vi "HFRR ADV v07.vi"() -> ()   [LabVIEW 2025] (continued)
            n1283 = local read "TEMP"() -> (w1608:dbl)
            n1284 = local write "FF 3"(w1604) -> ()
            n1285 = Compound Arithmetic op=OR("FRICVALZ 4", "FRICVALZ 3", "FRICVALZ 2") -> (w1601:bool)
            n1286 = case shown="True" w1601 {
              tunnel: w1594 -> [_ w1615]
              frame False {
              }
              frame True {
                w1614 = FALSE ("FRICVALZ")
                n1287 = local write "FRICVALZ 3"(w1614) -> ()
                n1288 = local write "FRICVALZ 2"(w1614) -> ()
                n1289 = local write "FRICVALZ 4"(w1614) -> ()
                "FRICVALZ" <- w1615
              }
            }
            n1290 = Not A Number/Path/Refnum?(number/path/refnum=w1608) -> (NaN/Path/Refnum?=w1607:bool)
            n1291 = Not A Number/Path/Refnum?(number/path/refnum=w1604) -> (NaN/Path/Refnum?=w1606:bool)
            n1292 = Divide(x=w1604, y=1.96) -> (x/y=w1591:dbl)
            n1293 = Compound Arithmetic op=OR(w1607, w1606) -> (w1605:bool)
            n1294 = Not A Number/Path/Refnum?(number/path/refnum=w1591) -> (NaN/Path/Refnum?=w1602:bool)
            n1295 = case shown="True" w1605 {
              frame False {
              }
              frame True {
                n1296 = local write "TEMP"(0.0 ("TEMP")) -> ()
                n1297 = local write "FF 2"(0.0 ("FF 2")) -> ()
                n1298 = local write "reinit"(TRUE ("reinit")) -> ()
              }
            }
            n1299 = Select(t=0.0, s=w1602, f=w1591) -> (s? t:f=w1590:dbl)
            "COF 2" <- w1590
            n1300 = local write "COF 3"(w1590) -> ()
          }
        }
      }
    }
    n1301 = Wait (ms)(milliseconds to wait=u32 50) -> ()  [unwired: 1 out]
    n1302 = local read "Quit"() -> (w1530:bool)
    "Rate" <- 2500.0 ("No of Samples")
  }
  n1303 = VISA Close(VISA resource name=w52, error in (no error)=w51) -> (error out=w49:errorcluster)
  n1304 = call <vilib>:"Clear Errors.vi"("error in (no error)"=w49) -> ()  [unwired: 5 in, 2 out]
  n1305 = VISA Close(VISA resource name=w37, error in (no error)=w36) -> ()  [unwired: 1 out]
  n1306 = while {
    tunnel: w57 -> [_]
    tunnel: [w1642] -> _
    tunnel: [w1618] -> w56
    i -> [w1642]
    stop <- w1618 stop-if-true
    # "C:\\LAB-IQ-NXT\\Scar View.exe"
    n1307 = local read "OK Button 16"() -> (w1631:bool)
    n1308 = local read "Main Tab"() -> (w1624:T2)
    n1309 = local read "service 3"() -> (w1625:bool)
    n1310 = local read "OPEN 6"() -> (w1627:bool)
    n1311 = local read "EDIT 2"() -> (w1629:bool)
    n1312 = local read "RUN"() -> (w1639:bool)
    n1313 = local read "RUN"() -> (w1641:bool)
    n1314 = case shown="True" "EDIT 3" {
      frame False {
      }
      frame True {
        n1315 = local write "EDIT 3"(FALSE ("EDIT 3")) -> ()
        n1316 = local write "Main Tab"(T2."About" ("Main Tab")) -> ()
      }
    }
    n1317 = case shown="\"CEC F-096-A-06\"" "TEST STANDARD" {
      tunnel: [2.0 ("Set Temp") 0.0 ("Set Temp") 2.0 ("Set Temp") 0.0 ("Set Temp")] -> w1630
      frame "ASTM D6079", Default {
        w2183 = 50.0 ("Hz")
        w2184 = 53.0 ("Set Rh")
        w2186 = 1.0 ("Set Strk")
        w2185 = 60.0 ("Set Temp")
        # "astm hide"
        n1318 = local write "NORMAL LOAD"(200.0 ("NORMAL LOAD")) -> ()
        n1319 = local write "Set Strk"(w2186) -> ()
        n1320 = local write "Set Hz"(w2183) -> ()
        n1321 = local write "test time"(75.0 ("test time")) -> ()
        n1322 = local write "Set Rh"(w2184) -> ()
        n1323 = local write "Set Temp"(w2185) -> ()
        n1324 = local write "Set Stroke:"(w2186) -> ()
        n1325 = local write "Set Humidity:"(w2184) -> ()
        n1326 = local write "Set Frequency:"(w2183) -> ()
        n1327 = local write "Set Temperature:"(w2185) -> ()
        "Test Standard" <- "ASTM D6079" ("Test Standard 2")
      }
      frame "ISO 12156" {
        n1328 = local write "NORMAL LOAD"(200.0 ("NORMAL LOAD")) -> ()
        n1329 = local write "Set Strk"(1.0 ("Set Strk")) -> ()
        n1330 = local write "Set Hz"(50.0 ("Hz")) -> ()
        n1331 = local write "test time"(75.0 ("test time")) -> ()
        n1332 = local write "Set Rh"(53.0 ("Set Rh")) -> ()
        n1333 = local write "Set Temp"(60.0 ("Set Temp")) -> ()
      }
      frame "CEC F-096-A-06" {
        n1334 = local write "NORMAL LOAD"(200.0 ("NORMAL LOAD")) -> ()
        n1335 = local write "Set Strk"(1.0 ("Set Strk")) -> ()
        n1336 = local write "Set Hz"(50.0 ("Hz")) -> ()
        n1337 = local write "test time"(75.0 ("test time")) -> ()
        n1338 = local write "Set Rh"(53.0 ("Set Rh")) -> ()
        n1339 = local write "Set Temp"(60.0 ("Set Temp")) -> ()
      }
      frame "Custom" {
      }
    }
    n1340 = case shown="False" w1639 {
      frame False {
      }
      frame True {
      }
    }
    n1341 = Or(x=w1627, y=w1625) -> (x .or. y?=w1626:bool)
    n1342 = case shown="\"About\"" w1624 {
      tunnel: [T23."Acquire" ("Main Tab") T23."Compare Files" ("Main Tab") T23."About" ("Main Tab")] -> w1637
      frame "Acquire", Default {
      }
      frame "Compare Files" {
      }
      frame "About" {
      }
    }
    n1343 = Or(x=w1631, y="OPEN") -> (x .or. y?=w1632:bool)
    n1344 = case shown="True" w1632 {
      tunnel: w1631 -> [_ w1772]
      frame False {
      }
      frame True {
        n1345 = stacked-sequence {
          tunnel: w1772 -> [_ w1839 _ _]
          frame #0 {
            w1788 = "  " ("String 6")
            n1346 = local write "OPEN"(FALSE ("open")) -> ()
            n1347 = local read "string1 4"() -> (w1774:string)
            n1348 = local read "string1 3"() -> (w1775:string)
            n1349 = local read "string1 2"() -> (w1776:string)
            n1350 = local write "String 6"(w1788) -> ()
            n1351 = local write "String 7"(w1788) -> ()
            n1352 = local write "String 8"(w1788) -> ()
            n1353 = local write "String 12"(w1788) -> ()
            n1354 = property on="OPEN" class="Bool (strict)"("Visible"=FALSE) -> ()  [unwired: 2 in, 2 out]
            n1355 = local read "OK Button 16"() -> (w1773:bool)
            n1356 = String To Path(string=w1774) -> (path=w1782:path)
            n1357 = String To Path(string=w1775) -> (path=w1783:path)
            n1358 = String To Path(string=w1776) -> (path=w1784:path)
            n1359 = case shown="True" w1773 {
              tunnel: [w1789 w1790] -> w1777
              frame False {
                n1360 = local read "string1"() -> (w1789:string)
              }
              frame True {
                n1361 = local read "String Indicator 4"() -> (w1790:string)
              }
            }
            n1362 = Open/Create/Replace File "Open File"(file path (use dialog)=w1784) -> (refnum out=w1780:refnum<file>)  [unwired: 5 in, 2 out]
            n1363 = Open/Create/Replace File "Open File"(file path (use dialog)=w1783) -> (refnum out=w1779:refnum<file>)  [unwired: 5 in, 2 out]
            n1364 = Open/Create/Replace File "Open File"(file path (use dialog)=w1782) -> (refnum out=w1778:refnum<file>)  [unwired: 5 in, 2 out]
            n1365 = while {
              tunnel: w1780 -> [w1802]
              i -> [w1798]
              stop <- w1797 continue-if-true
              (unwired) TRUE ("line mode (F)")
              n1366 = Read from Text File "Read File"(file (use dialog)=w1802) -> (text=w1799:string)  [unwired: 3 in, 3 out]
              n1367 = local write "Numeric 11"(w1798) -> ()
              n1368 = String Length(string=w1799) -> (length=w1801:i32)
              n1369 = Greater?(x=w1801, y=1) -> (0:w1797:bool)
            }
            n1370 = while {
              tunnel: w1779 -> [w1808]
              i -> [w1804]
              stop <- w1803 continue-if-true
              (unwired) TRUE ("line mode (F)")
              n1371 = Read from Text File "Read File"(file (use dialog)=w1808) -> (text=w1805:string)  [unwired: 3 in, 3 out]
              n1372 = local write "Numeric 12"(w1804) -> ()
              n1373 = String Length(string=w1805) -> (length=w1807:i32)
              n1374 = Greater?(x=w1807, y=1) -> (0:w1803:bool)
            }
            n1375 = while {
              tunnel: w1778 -> [w1814]
              i -> [w1810]
              stop <- w1809 continue-if-true
              (unwired) TRUE ("line mode (F)")
              n1376 = Read from Text File "Read File"(file (use dialog)=w1814) -> (text=w1811:string)  [unwired: 3 in, 3 out]
              n1377 = local write "Numeric 13"(w1810) -> ()
              n1378 = String Length(string=w1811) -> (length=w1813:i32)
              n1379 = Greater?(x=w1813, y=1) -> (0:w1809:bool)
            }
            n1380 = String To Path(string=w1777) -> (path=w1785:path)
            n1381 = Open/Create/Replace File "Open File"(file path (use dialog)=w1785) -> (refnum out=w1781:refnum<file>)  [unwired: 5 in, 2 out]
            n1382 = while {
              tunnel: w1781 -> [w1796]
              i -> [w1792]
              stop <- w1791 continue-if-true
              (unwired) TRUE ("line mode (F)")
              n1383 = Read from Text File "Read File"(file (use dialog)=w1796) -> (text=w1793:string)  [unwired: 3 in, 3 out]
              n1384 = local write "Numeric 8"(w1792) -> ()
              n1385 = String Length(string=w1793) -> (length=w1795:i32)
              n1386 = Greater?(x=w1795, y=1) -> (0:w1791:bool)
            }
          }
          frame #1 {
            w1966 = FALSE ("ACTUAL   MERGE")
            # "Sample Temp"
            # "ECR"
            # "COF"
            # "Time\nCOF\nFF\nTemp"
            n1387 = case shown="True" w1839 {
              tunnel: [w1986 w1987] -> w1840
              frame False {
                n1388 = local read "string1"() -> (w1986:string)
              }
              frame True {
                n1389 = local read "String Indicator 4"() -> (w1987:string)
              }
            }
            n1390 = local read "string1 3"() -> (w1884:string)
            n1391 = String To Path(string=w1884) -> (path=w1982:path)
            n1392 = String To Path(string=w1840) -> (path=w1971:path)
            n1393 = local read "Numeric 12"() -> (w1968:i32)
            n1394 = local read "Numeric 8"() -> (w1970:i32)
            n1395 = local read "string1 4"() -> (w1883:string)
            n1396 = local read "string1 2"() -> (w1885:string)
            n1397 = Open/Create/Replace File "Open File"(file path (use dialog)=w1971) -> (refnum out=w1985:refnum<file>, error out=w1984:errorcluster)  [unwired: 5 in, 1 out]
            n1398 = Open/Create/Replace File "Open File"(file path (use dialog)=w1982) -> (refnum out=w1978:refnum<file>, error out=w1979:errorcluster)  [unwired: 5 in, 1 out]
            n1399 = for {
              N: w1968 -> [_]
              tunnel: w1979 -> [w2059]
              tunnel: w1978 -> [w2058]
              tunnel: [w2048] -> w1937 mode=indexing
              tunnel: [w2046] -> w1935 mode=indexing
              tunnel: [w2047] -> w1931 mode=indexing
              tunnel: w1966 -> [_]
              tunnel: [w2040] -> w1933 mode=indexing
              tunnel: [w2036] -> w1915 mode=indexing
              tunnel: [w2032] -> w1891 mode=indexing
              tunnel: [w2029] -> w1872 mode=indexing
              tunnel: [w2025] -> w1831 mode=indexing
              (unwired) 9 ("length (rest)")
              (unwired) 9 ("length (rest)")
              (unwired) TRUE ("line mode (F)")
              n1400 = Read from Text File "Read File"(file (use dialog)=w2058, error in=w2059) -> (text=w2026:string)  [unwired: 2 in, 3 out]
              n1401 = local write "String 8"(w2026) -> ()
              n1402 = String Subset(string=w2026, offset (0)=85) -> (substring=w2028:string)  [unwired: 1 in]
              n1403 = String Subset(string=w2026, offset (0)=25) -> (substring=w2030:string)  [unwired: 1 in]
              n1404 = String Subset(string=w2026, offset (0)=55, length (rest)=9 ("length (rest)")) -> (substring=w2034:string)
              n1405 = String Subset(string=w2026, offset (0)=45, length (rest)=9 ("length (rest)")) -> (substring=w2039:string)
              n1406 = String Subset(string=w2026, offset (0)=65, length (rest)=9 ("length (rest)")) -> (substring=w2045:string)
              n1407 = String Subset(string=w2026, offset (0)=35, length (rest)=9 ("length (rest)")) -> (substring=w2049:string)
              n1408 = String Subset(string=w2026, offset (0)=0, length (rest)=14 ("length (rest)")) -> (substring=w2052:string)
              n1409 = String Subset(string=w2026, offset (0)=15, length (rest)=9 ("length (rest)")) -> (substring=w2055:string)
              n1410 = Fract/Exp String To Number(string=w2028) -> (number=w2025:dbl)  [unwired: 3 in, 1 out]
              n1411 = Fract/Exp String To Number(string=w2030) -> (number=w2029:dbl)  [unwired: 3 in, 1 out]
              n1412 = Fract/Exp String To Number(string=w2034) -> (number=w2032:dbl)  [unwired: 3 in, 1 out]
              n1413 = Fract/Exp String To Number(string=w2039) -> (number=w2036:dbl)  [unwired: 3 in, 1 out]
              n1414 = Fract/Exp String To Number(string=w2045) -> (number=w2042:dbl)  [unwired: 3 in, 1 out]
              n1415 = Fract/Exp String To Number(string=w2049) -> (number=w2047:dbl)  [unwired: 3 in, 1 out]
              n1416 = Fract/Exp String To Number(string=w2052) -> (number=w2048:dbl)  [unwired: 3 in, 1 out]
              n1417 = Fract/Exp String To Number(string=w2055) -> (number=w2046:dbl)  [unwired: 3 in, 1 out]
              n1418 = Add(x=w2042, y=0.0) -> (x+y=w2040:dbl)
            }
            n1419 = for {
              N: w1970 -> [_]
              tunnel: w1985 -> [w2133]
              tunnel: w1984 -> [w2132]
              tunnel: [w2122] -> w1897 mode=indexing
              tunnel: [w2120] -> w1954 mode=indexing
              tunnel: [w2121] -> w1949 mode=indexing
              tunnel: w1966 -> [_]
              tunnel: [w2114] -> w1951 mode=indexing
              tunnel: [w2110] -> w1920 mode=indexing
              tunnel: [w2106] -> w1895 mode=indexing
              tunnel: [w2102] -> w1876 mode=indexing
              tunnel: [w2097] -> w1836 mode=indexing
              (unwired) TRUE ("line mode (F)")
              # "freq"
              # "Stroke"
              # "Time"
              # "CoF"
              # "Humidity"
              # "Temp"
              # "Air Temp"
              # "ECR"
              n1420 = Read from Text File "Read File"(file (use dialog)=w2133, error in=w2132) -> (text=w2098:string)  [unwired: 2 in, 3 out]
              n1421 = local write "String 6"(w2098) -> ()
              n1422 = String Subset(string=w2098, offset (0)=35, length (rest)=9 ("length (rest)")) -> (substring=w2123:string)
              n1423 = String Subset(string=w2098, offset (0)=0, length (rest)=14 ("length (rest)")) -> (substring=w2126:string)
              n1424 = String Subset(string=w2098, offset (0)=15, length (rest)=9 ("length (rest)")) -> (substring=w2129:string)
              n1425 = Fract/Exp String To Number(string=w2123) -> (number=w2121:dbl)  [unwired: 3 in, 1 out]
              n1426 = Fract/Exp String To Number(string=w2126) -> (number=w2122:dbl)  [unwired: 3 in, 1 out]
              n1427 = Fract/Exp String To Number(string=w2129) -> (number=w2120:dbl)  [unwired: 3 in, 1 out]
              n1428 = String Subset(string=w2098, offset (0)=85, length (rest)=9 ("length (rest)")) -> (substring=w2099:string)
              n1429 = String Subset(string=w2098, offset (0)=25, length (rest)=9 ("length (rest)")) -> (substring=w2105:string)
              n1430 = String Subset(string=w2098, offset (0)=55, length (rest)=9 ("length (rest)")) -> (substring=w2107:string)
              n1431 = String Subset(string=w2098, offset (0)=45, length (rest)=9 ("length (rest)")) -> (substring=w2113:string)
              n1432 = String Subset(string=w2098, offset (0)=65, length (rest)=9 ("length (rest)")) -> (substring=w2119:string)
              n1433 = Fract/Exp String To Number(string=w2105) -> (number=w2102:dbl)  [unwired: 3 in, 1 out]
              n1434 = Fract/Exp String To Number(string=w2099) -> (number=w2097:dbl)  [unwired: 3 in, 1 out]
              n1435 = Fract/Exp String To Number(string=w2107) -> (number=w2106:dbl)  [unwired: 3 in, 1 out]
              n1436 = Fract/Exp String To Number(string=w2113) -> (number=w2110:dbl)  [unwired: 3 in, 1 out]
              n1437 = Fract/Exp String To Number(string=w2119) -> (number=w2116:dbl)  [unwired: 3 in, 1 out]
              n1438 = Add(x=w2116, y=0.0) -> (x+y=w2114:dbl)
            }
            n1439 = String To Path(string=w1883) -> (path=w1977:path)
            n1440 = String To Path(string=w1885) -> (path=w1983:path)
            n1441 = local read "Numeric 11"() -> (w1967:i32)
            n1442 = local read "Numeric 13"() -> (w1969:i32)
            n1443 = Open/Create/Replace File "Open File"(file path (use dialog)=w1983) -> (refnum out=w1981:refnum<file>, error out=w1980:errorcluster)  [unwired: 5 in, 1 out]
            n1444 = Open/Create/Replace File "Open File"(file path (use dialog)=w1977) -> (refnum out=w1976:refnum<file>, error out=w1975:errorcluster)  [unwired: 5 in, 1 out]
            n1445 = for {
              N: w1969 -> [_]
              tunnel: w1976 -> [w2024]
              tunnel: w1975 -> [w2023]
              tunnel: [w2013] -> w1929 mode=indexing
              tunnel: [w2012] -> w1922 mode=indexing
              tunnel: w1966 -> [_]
              tunnel: [w2001] -> w1927 mode=indexing
              tunnel: [w2006] -> w1924 mode=indexing
              tunnel: [w2002] -> w1914 mode=indexing
              tunnel: [w1997] -> w1889 mode=indexing
              tunnel: [w1993] -> w1870 mode=indexing
              tunnel: [w1988] -> w1830 mode=indexing
              (unwired) 1.0 ("x")
              (unwired) TRUE ("line mode (F)")
              n1446 = Read from Text File "Read File"(file (use dialog)=w2024, error in=w2023) -> (text=w1989:string)  [unwired: 2 in, 3 out]
              n1447 = local write "String 12"(w1989) -> ()
              n1448 = String Subset(string=w1989, offset (0)=85, length (rest)=9 ("length (rest)")) -> (substring=w1991:string)
              n1449 = String Subset(string=w1989, offset (0)=25, length (rest)=9 ("length (rest)")) -> (substring=w1995:string)
              n1450 = String Subset(string=w1989, offset (0)=55, length (rest)=9 ("length (rest)")) -> (substring=w1999:string)
              n1451 = String Subset(string=w1989, offset (0)=45, length (rest)=9 ("length (rest)")) -> (substring=w2004:string)
              n1452 = String Subset(string=w1989, offset (0)=65, length (rest)=9 ("length (rest)")) -> (substring=w2007:string)
              n1453 = String Subset(string=w1989, offset (0)=35, length (rest)=9 ("length (rest)")) -> (substring=w2014:string)
              n1454 = String Subset(string=w1989, offset (0)=0, length (rest)=14 ("length (rest)")) -> (substring=w2017:string)
              n1455 = String Subset(string=w1989, offset (0)=15, length (rest)=9 ("length (rest)")) -> (substring=w2020:string)
              n1456 = Fract/Exp String To Number(string=w1991) -> (number=w1988:dbl)  [unwired: 3 in, 1 out]
              n1457 = Fract/Exp String To Number(string=w1995) -> (number=w1993:dbl)  [unwired: 3 in, 1 out]
              n1458 = Fract/Exp String To Number(string=w1999) -> (number=w1997:dbl)  [unwired: 3 in, 1 out]
              n1459 = Fract/Exp String To Number(string=w2004) -> (number=w2002:dbl)  [unwired: 3 in, 1 out]
              n1460 = Fract/Exp String To Number(string=w2007) -> (number=w2010:dbl)  [unwired: 3 in, 1 out]
              n1461 = Fract/Exp String To Number(string=w2014) -> (number=w2012:dbl)  [unwired: 3 in, 1 out]
              n1462 = Fract/Exp String To Number(string=w2017) -> (number=w2013:dbl)  [unwired: 3 in, 1 out]
              n1463 = Fract/Exp String To Number(string=w2020) -> (number=w2001:dbl)  [unwired: 3 in, 1 out]
              n1464 = Add(x=w2010, y=0.0) -> (x+y=w2006:dbl)
            }
            n1465 = for {
              N: w1967 -> [_]
              tunnel: w1981 -> [w2096]
              tunnel: w1980 -> [w2095]
              tunnel: [w2085] -> w1947 mode=indexing
              tunnel: [w2083] -> w1945 mode=indexing
              tunnel: [w2084] -> w1940 mode=indexing
              tunnel: w1966 -> [_]
              tunnel: [w2077] -> w1942 mode=indexing
              tunnel: [w2073] -> w1918 mode=indexing
              tunnel: [w2069] -> w1893 mode=indexing
              tunnel: [w2065] -> w1874 mode=indexing
              tunnel: [w2060] -> w1832 mode=indexing
              (unwired) TRUE ("line mode (F)")
              n1466 = Read from Text File "Read File"(file (use dialog)=w2096, error in=w2095) -> (text=w2061:string)  [unwired: 2 in, 3 out]
              n1467 = local write "String 7"(w2061) -> ()
              n1468 = String Subset(string=w2061, offset (0)=85, length (rest)=9 ("length (rest)")) -> (substring=w2064:string)
              n1469 = String Subset(string=w2061, offset (0)=25, length (rest)=9 ("length (rest)")) -> (substring=w2066:string)
              n1470 = String Subset(string=w2061, offset (0)=55, length (rest)=9 ("length (rest)")) -> (substring=w2072:string)
              n1471 = String Subset(string=w2061, offset (0)=45, length (rest)=9 ("length (rest)")) -> (substring=w2074:string)
              n1472 = String Subset(string=w2061, offset (0)=65, length (rest)=9 ("length (rest)")) -> (substring=w2078:string)
              n1473 = String Subset(string=w2061, offset (0)=35, length (rest)=9 ("length (rest)")) -> (substring=w2086:string)
              n1474 = String Subset(string=w2061, offset (0)=0, length (rest)=14 ("length (rest)")) -> (substring=w2089:string)
              n1475 = String Subset(string=w2061, offset (0)=15, length (rest)=9 ("length (rest)")) -> (substring=w2092:string)
              n1476 = Fract/Exp String To Number(string=w2064) -> (number=w2060:dbl)  [unwired: 3 in, 1 out]
              n1477 = Fract/Exp String To Number(string=w2066) -> (number=w2065:dbl)  [unwired: 3 in, 1 out]
              n1478 = Fract/Exp String To Number(string=w2072) -> (number=w2069:dbl)  [unwired: 3 in, 1 out]
              n1479 = Fract/Exp String To Number(string=w2074) -> (number=w2073:dbl)  [unwired: 3 in, 1 out]
              n1480 = Fract/Exp String To Number(string=w2078) -> (number=w2081:dbl)  [unwired: 3 in, 1 out]
              n1481 = Fract/Exp String To Number(string=w2086) -> (number=w2084:dbl)  [unwired: 3 in, 1 out]
              n1482 = Fract/Exp String To Number(string=w2089) -> (number=w2085:dbl)  [unwired: 3 in, 1 out]
              n1483 = Fract/Exp String To Number(string=w2092) -> (number=w2083:dbl)  [unwired: 3 in, 1 out]
              n1484 = Add(x=w2081, y=0.0) -> (x+y=w2077:dbl)
            }
            n1485 = Delete From Array(array=w1872, index=0) -> (array with subset deleted=w1845:dbl[])  [unwired: 1 in, 1 out]
            n1486 = Delete From Array(array=w1915, index=0) -> (array with subset deleted=w1903:dbl[])  [unwired: 1 in, 1 out]
            n1487 = Delete From Array(array=w1933, index=0) -> (array with subset deleted=w1934:dbl[])  [unwired: 1 in, 1 out]
            n1488 = Delete From Array(array=w1935, index=0) -> (array with subset deleted=w1908:dbl[])  [unwired: 1 in, 1 out]
            n1489 = call-poly <vilib>:"Mean.vi"("X"=w1908) -> ("mean"=→"КОФ3":dbl)  [unwired: 1 out]
            n1490 = call-poly <vilib>:"Mean.vi"("X"=w1903) -> ("mean"=→"CP3":dbl)  [unwired: 1 out]
            n1491 = call-poly <vilib>:"Mean.vi"("X"=w1845) -> ("mean"=→"КОФ2 4":dbl)  [unwired: 1 out]
            n1492 = Delete From Array(array=w1836, index=0) -> (array with subset deleted=w1823:dbl[])  [unwired: 1 in, 1 out]
            n1493 = Delete From Array(array=w1876, index=0) -> (array with subset deleted=w1847:dbl[])  [unwired: 1 in, 1 out]
            n1494 = Delete From Array(array=w1920, index=0) -> (array with subset deleted=w1905:dbl[])  [unwired: 1 in, 1 out]
            "array w/ subset deleted" <- w1905
            n1495 = Delete From Array(array=w1951, index=0) -> (array with subset deleted=w1952:dbl[])  [unwired: 1 in, 1 out]
            n1496 = Delete From Array(array=w1954, index=0) -> (array with subset deleted=w1909:dbl[])  [unwired: 1 in, 1 out]
            n1497 = Delete From Array(array=w1897, index=0) -> (array with subset deleted=w1824:dbl[])  [unwired: 1 in, 1 out]
            n1498 = call-poly <vilib>:"Mean.vi"("X"=w1909) -> ("mean"=→"КОФ1":dbl)  [unwired: 1 out]
            n1499 = call-poly <vilib>:"Mean.vi"("X"=w1847) -> ("mean"=→"КОФ2 2":dbl)  [unwired: 1 out]
            n1500 = Bundle "Bundle"(w1824, w1823) -> (w1829:cluster{dbl[], dbl[]})  [unwired: 1 in]
            n1501 = Bundle "Bundle"(w1824, w1952) -> (w1816:cluster{dbl[], dbl[]})  [unwired: 1 in]
            n1502 = Delete From Array(array=w1830, index=0) -> (array with subset deleted=w1817:dbl[])  [unwired: 1 in, 1 out]
            n1503 = Delete From Array(array=w1831, index=0) -> (array with subset deleted=w1819:dbl[])  [unwired: 1 in, 1 out]
            n1504 = Delete From Array(array=w1832, index=0) -> (array with subset deleted=w1821:dbl[])  [unwired: 1 in, 1 out]
            n1505 = Delete From Array(array=w1924, index=0) -> (array with subset deleted=w1925:dbl[])  [unwired: 1 in, 1 out]
            n1506 = Delete From Array(array=w1942, index=0) -> (array with subset deleted=w1943:dbl[])  [unwired: 1 in, 1 out]
            n1507 = Delete From Array(array=w1870, index=0) -> (array with subset deleted=w1844:dbl[])  [unwired: 1 in, 1 out]
            n1508 = Delete From Array(array=w1874, index=0) -> (array with subset deleted=w1846:dbl[])  [unwired: 1 in, 1 out]
            n1509 = Delete From Array(array=w1889, index=0) -> (array with subset deleted=w1848:dbl[])  [unwired: 1 in, 1 out]
            n1510 = Delete From Array(array=w1891, index=0) -> (array with subset deleted=w1849:dbl[])  [unwired: 1 in, 1 out]
            n1511 = Delete From Array(array=w1893, index=0) -> (array with subset deleted=w1850:dbl[])  [unwired: 1 in, 1 out]
            n1512 = Delete From Array(array=w1895, index=0) -> (array with subset deleted=w1851:dbl[])  [unwired: 1 in, 1 out]
            n1513 = Delete From Array(array=w1914, index=0) -> (array with subset deleted=w1902:dbl[])  [unwired: 1 in, 1 out]
            n1514 = Delete From Array(array=w1918, index=0) -> (array with subset deleted=w1904:dbl[])  [unwired: 1 in, 1 out]
            n1515 = Delete From Array(array=w1922, index=0) -> (array with subset deleted=w1852:dbl[])  [unwired: 1 in, 1 out]
            n1516 = Delete From Array(array=w1927, index=0) -> (array with subset deleted=w1907:dbl[])  [unwired: 1 in, 1 out]
            n1517 = Delete From Array(array=w1931, index=0) -> (array with subset deleted=w1853:dbl[])  [unwired: 1 in, 1 out]
            n1518 = Delete From Array(array=w1940, index=0) -> (array with subset deleted=w1854:dbl[])  [unwired: 1 in, 1 out]
            n1519 = Delete From Array(array=w1945, index=0) -> (array with subset deleted=w1906:dbl[])  [unwired: 1 in, 1 out]
            n1520 = Delete From Array(array=w1949, index=0) -> (array with subset deleted=w1855:dbl[])  [unwired: 1 in, 1 out]
            n1521 = Delete From Array(array=w1929, index=0) -> (array with subset deleted=w1818:dbl[])  [unwired: 1 in, 1 out]
            n1522 = Delete From Array(array=w1937, index=0) -> (array with subset deleted=w1820:dbl[])  [unwired: 1 in, 1 out]
            n1523 = Delete From Array(array=w1947, index=0) -> (array with subset deleted=w1822:dbl[])  [unwired: 1 in, 1 out]
            n1524 = Bundle "Bundle"(w1818, w1817) -> (w1826:cluster{dbl[], dbl[]})  [unwired: 1 in]
            n1525 = Bundle "Bundle"(w1820, w1819) -> (w1827:cluster{dbl[], dbl[]})  [unwired: 1 in]
            n1526 = Bundle "Bundle"(w1822, w1821) -> (w1828:cluster{dbl[], dbl[]})  [unwired: 1 in]
            n1527 = Bundle "Bundle"(w1852, w1848) -> (w1860:cluster{dbl[], dbl[]})  [unwired: 1 in]
            n1528 = Bundle "Bundle"(w1853, w1849) -> (w1859:cluster{dbl[], dbl[]})  [unwired: 1 in]
            n1529 = Bundle "Bundle"(w1854, w1850) -> (w1858:cluster{dbl[], dbl[]})  [unwired: 1 in]
            n1530 = Bundle "Bundle"(w1855, w1851) -> (w1857:cluster{dbl[], dbl[]})  [unwired: 1 in]
            n1531 = Bundle "Bundle"(w1818, w1848) -> (w1886:cluster{dbl[], dbl[]})  [unwired: 1 in]
            n1532 = Bundle "Bundle"(w1820, w1849) -> (w1887:cluster{dbl[], dbl[]})  [unwired: 1 in]
            n1533 = Bundle "Bundle"(w1822, w1850) -> (w1888:cluster{dbl[], dbl[]})  [unwired: 1 in]
            n1534 = Bundle "Bundle"(w1818, w1902) -> (w1910:cluster{dbl[], dbl[]})  [unwired: 1 in]
            n1535 = Bundle "Bundle"(w1820, w1903) -> (w1911:cluster{dbl[], dbl[]})  [unwired: 1 in]
            n1536 = Bundle "Bundle"(w1822, w1904) -> (w1912:cluster{dbl[], dbl[]})  [unwired: 1 in]
            n1537 = Bundle "Bundle"(w1822, w1943) -> (w1956:cluster{dbl[], dbl[]})  [unwired: 1 in]
            n1538 = Bundle "Bundle"(w1820, w1934) -> (w1958:cluster{dbl[], dbl[]})  [unwired: 1 in]
            n1539 = Bundle "Bundle"(w1818, w1925) -> (w1957:cluster{dbl[], dbl[]})  [unwired: 1 in]
            n1540 = Bundle "Bundle"(w1824, w1855) -> (w1842:cluster{dbl[], dbl[]})  [unwired: 1 in]
            n1541 = Bundle "Bundle"(w1822, w1854) -> (w1965:cluster{dbl[], dbl[]})  [unwired: 1 in]
            n1542 = Bundle "Bundle"(w1820, w1853) -> (w1963:cluster{dbl[], dbl[]})  [unwired: 1 in]
            n1543 = Bundle "Bundle"(w1818, w1852) -> (w1964:cluster{dbl[], dbl[]})  [unwired: 1 in]
            n1544 = Bundle "Bundle"(w1824, w1909) -> (w1843:cluster{dbl[], dbl[]})  [unwired: 1 in]
            n1545 = Bundle "Bundle"(w1822, w1906) -> (w1974:cluster{dbl[], dbl[]})  [unwired: 1 in]
            n1546 = Bundle "Bundle"(w1820, w1908) -> (w1973:cluster{dbl[], dbl[]})  [unwired: 1 in]
            n1547 = Bundle "Bundle"(w1818, w1907) -> (w1972:cluster{dbl[], dbl[]})  [unwired: 1 in]
            n1548 = call-poly <vilib>:"Mean.vi"("X"=w1906) -> ("mean"=→"КОФ2":dbl)  [unwired: 1 out]
            n1549 = call-poly <vilib>:"Mean.vi"("X"=w1907) -> ("mean"=→"КОФ4":dbl)  [unwired: 1 out]
            n1550 = call-poly <vilib>:"Mean.vi"("X"=w1905) -> ("mean"=→"CP1":dbl)  [unwired: 1 out]
            n1551 = call-poly <vilib>:"Mean.vi"("X"=w1904) -> ("mean"=→"CP2":dbl)  [unwired: 1 out]
            n1552 = call-poly <vilib>:"Mean.vi"("X"=w1902) -> ("mean"=→"CP4":dbl)  [unwired: 1 out]
            n1553 = call-poly <vilib>:"Mean.vi"("X"=w1846) -> ("mean"=→"КОФ2 3":dbl)  [unwired: 1 out]
            n1554 = call-poly <vilib>:"Mean.vi"("X"=w1844) -> ("mean"=→"КОФ2 5":dbl)  [unwired: 1 out]
            n1555 = Bundle "Bundle"(w1824, w1851) -> (w1815:cluster{dbl[], dbl[]})  [unwired: 1 in]
            n1556 = Bundle "Bundle"(w1824, w1905) -> (w1838:cluster{dbl[], dbl[]})  [unwired: 1 in]
            n1557 = Build Array "Build Array"(w1829, w1828, w1827, w1826) -> (→"Frequency ( Hz )":cluster{dbl[], dbl[]}[])
            n1558 = Build Array "Build Array"(w1815, w1838) -> (w1841:cluster{dbl[], dbl[]}[])
            "XY Graph 17" <- w1841
            n1559 = Build Array "Build Array"(w1857, w1858, w1859, w1860) -> (→"Air Temp ( °C ) vs Humidity ( % RH )":cluster{dbl[], dbl[]}[])
            n1560 = Build Array "Build Array"(w1815, w1888, w1887, w1886) -> (→"Humidity ( %RH )":cluster{dbl[], dbl[]}[])
            n1561 = Build Array "Build Array"(w1838, w1912, w1911, w1910) -> (→"Sample Temperature ( °C )":cluster{dbl[], dbl[]}[])
            n1562 = Build Array "Build Array"(w1816, w1956, w1958, w1957) -> (→"XY Graph 13":cluster{dbl[], dbl[]}[])
            n1563 = Build Array "Build Array"(w1842, w1965, w1963, w1964) -> (→"Air Temperature  ( °C )":cluster{dbl[], dbl[]}[])
            n1564 = Build Array "Build Array"(w1843, w1974, w1973, w1972) -> (→"Coefficient Of Friction":cluster{dbl[], dbl[]}[])
            n1565 = Bundle "Bundle"(w1818, w1844) -> (w1866:cluster{dbl[], dbl[]})  [unwired: 1 in]
            n1566 = Bundle "Bundle"(w1820, w1845) -> (w1867:cluster{dbl[], dbl[]})  [unwired: 1 in]
            n1567 = Bundle "Bundle"(w1822, w1846) -> (w1868:cluster{dbl[], dbl[]})  [unwired: 1 in]
            n1568 = Bundle "Bundle"(w1824, w1847) -> (w1869:cluster{dbl[], dbl[]})  [unwired: 1 in]
            n1569 = Build Array "Build Array"(w1869, w1868, w1867, w1866) -> (→"Stroke ( mm )":cluster{dbl[], dbl[]}[])
            n1570 = local write "XY Graph 16"(w1841) -> ()
          }
          frame #2 {
          }
          frame #3 {
            n1571 = local write "Numeric 8"(0 ("Numeric 8")) -> ()
            n1572 = local write "Numeric 11"(0 ("Numeric 11")) -> ()
            n1573 = local write "Numeric 12"(0 ("Numeric 12")) -> ()
            n1574 = local write "Numeric 13"(0 ("Numeric 13")) -> ()
            n1575 = property on="OPEN" class="Bool (strict)"("Visible"=TRUE) -> ()  [unwired: 2 in, 2 out]
            n1576 = local read "String Control 8"() -> (w2138:string)
            n1577 = local read "String Control 6"() -> (w2139:string)
            n1578 = local read "String Control 4"() -> (w2140:string)
            n1579 = local read "String Control 2"() -> (w2141:string)
            n1580 = Match Pattern(string=w2138, regular expression="Samples / cycle :- ") -> (after substring=w2143:string)  [unwired: 1 in, 3 out]
            n1581 = Match Pattern(string=w2139, regular expression="Samples / cycle :- ") -> (after substring=w2147:string)  [unwired: 1 in, 3 out]
            n1582 = Match Pattern(string=w2140, regular expression="Samples / cycle :- ") -> (after substring=w2151:string)  [unwired: 1 in, 3 out]
            n1583 = Match Pattern(string=w2141, regular expression="Samples / cycle :- ") -> (after substring=w2155:string)  [unwired: 1 in, 3 out]
            n1584 = Match Pattern(string=w2138, regular expression="Frequency :- ") -> (after substring=w2159:string)  [unwired: 1 in, 3 out]
            n1585 = Match Pattern(string=w2139, regular expression="Frequency :- ") -> (after substring=w2164:string)  [unwired: 1 in, 3 out]
            n1586 = Match Pattern(string=w2140, regular expression="Frequency :- ") -> (after substring=w2169:string)  [unwired: 1 in, 3 out]
            n1587 = Match Pattern(string=w2141, regular expression="Frequency :- ") -> (after substring=w2174:string)  [unwired: 1 in, 3 out]
            n1588 = String Subset(string=w2143, length (rest)=6 ("length (rest)")) -> (substring=w2145:string)  [unwired: 1 in]
            n1589 = String Subset(string=w2147, length (rest)=6 ("length (rest)")) -> (substring=w2149:string)  [unwired: 1 in]
            n1590 = String Subset(string=w2151, length (rest)=6 ("length (rest)")) -> (substring=w2153:string)  [unwired: 1 in]
            n1591 = String Subset(string=w2155, length (rest)=6 ("length (rest)")) -> (substring=w2157:string)  [unwired: 1 in]
            n1592 = String Subset(string=w2159, length (rest)=9 ("length (rest)")) -> (substring=w2161:string)  [unwired: 1 in]
            n1593 = String Subset(string=w2164, length (rest)=9 ("length (rest)")) -> (substring=w2166:string)  [unwired: 1 in]
            n1594 = String Subset(string=w2169, length (rest)=9 ("length (rest)")) -> (substring=w2171:string)  [unwired: 1 in]
            n1595 = String Subset(string=w2174, length (rest)=9 ("length (rest)")) -> (substring=w2176:string)  [unwired: 1 in]
            n1596 = Fract/Exp String To Number(string=w2145) -> (number=w2134:dbl)  [unwired: 3 in, 1 out]
            n1597 = Fract/Exp String To Number(string=w2149) -> (number=w2135:dbl)  [unwired: 3 in, 1 out]
            n1598 = Fract/Exp String To Number(string=w2153) -> (number=w2136:dbl)  [unwired: 3 in, 1 out]
            n1599 = Fract/Exp String To Number(string=w2157) -> (number=w2137:dbl)  [unwired: 3 in, 1 out]
            n1600 = Fract/Exp String To Number(string=w2161) -> (number=w2162:dbl)  [unwired: 3 in, 1 out]
            n1601 = Fract/Exp String To Number(string=w2166) -> (number=w2167:dbl)  [unwired: 3 in, 1 out]
            n1602 = Fract/Exp String To Number(string=w2171) -> (number=w2172:dbl)  [unwired: 3 in, 1 out]
            n1603 = Fract/Exp String To Number(string=w2176) -> (number=w2177:dbl)  [unwired: 3 in, 1 out]
            n1604 = local write "sample4"(w2134) -> ()
            n1605 = local write "sample3"(w2135) -> ()
            n1606 = local write "sample2"(w2136) -> ()
            n1607 = local write "sample1"(w2137) -> ()
            n1608 = local write "freq 4"(w2162) -> ()
            n1609 = local write "freq3"(w2167) -> ()
            n1610 = local write "freq2"(w2172) -> ()
            n1611 = local write "freq1"(w2177) -> ()
          }
        }
      }
    }
    n1612 = case shown="True" w1626 {
      selector: w1626 -> [_ w1754]
      frame False {
      }
      frame True {
        n1613 = Not(x=w1754) -> (.not. x?=w1750:bool)
        n1614 = local write "service 3"(w1750) -> ()
        n1615 = local write "OPEN 6"(w1750) -> ()
        n1616 = call <vilib>:"System Exec.vi"("wait until completion? (T)"=TRUE, "command line"="C:\\LAB-IQ\\Scar View.exe") -> ("error out"=→"error out 5":errorcluster)  [unwired: 6 in, 3 out]
      }
    }
    n1617 = flat-sequence {
      frame #0 {
        n1618 = local read "SAVE 2"() -> (w2244:bool)
        n1619 = local read "x = y?"() -> (w2250:bool)
        n1620 = local read "HUMIDITY: 2"() -> (w2252:dbl)
        n1621 = local read "HUMIDITY:"() -> (w2251:dbl)
        n1622 = case shown="True" "SrvM CP 2" {
          frame False {
          }
          frame True {
            n1623 = local write "SrvM CP 2"(FALSE ("SrvM CP 2")) -> ()
            n1624 = local read "HUMIDITY: 2"() -> (w2291:dbl)
            n1625 = local read "TEMP INTERCEPT: 2"() -> (w2290:dbl)
            n1626 = local read "DISPLACEMENT : 4"() -> (w2294:dbl)
            n1627 = local read "TEMPERATURE : 2"() -> (w2293:dbl)
            n1628 = local read "STROKE GAIN : 2"() -> (w2295:dbl)
            n1629 = local read "FRIC. FORCE : 2"() -> (w2296:dbl)
            n1630 = local read "AIR TEMP INTERCEPT: 2"() -> (w2289:dbl)
            n1631 = local read "AIR TEMPERATURE : 2"() -> (w2292:dbl)
            n1632 = local write "HUMIDITY:"(w2291) -> ()
            n1633 = local write "AIR TEMP INTERCEPT:"(w2290) -> ()
            n1634 = local write "TEMPERATURE :"(w2293) -> ()
            n1635 = local write "DISPLACEMENT :"(w2294) -> ()
            n1636 = local write "STROKE GAIN :"(w2295) -> ()
            n1637 = local write "FRIC. FORCE :"(w2296) -> ()
            n1638 = local write "TEMP INTERCEPT:"(w2289) -> ()
            n1639 = local write "AIR TEMPERATURE :"(w2292) -> ()
          }
        }
        n1640 = property on="Port 1 Error" class="Clust (strict)"("Visible"="EDIT") -> ()  [unwired: 2 in, 2 out]
        n1641 = property on="Port 2 Error" class="Clust (strict)"("Visible"="EDIT") -> ()  [unwired: 2 in, 2 out]
        n1642 = Or(x="SAVE", y=w2244) -> (x .or. y?=w2245:bool)
        n1643 = And(x="EDIT", y=w2250) -> (x .and. y?=w2248:bool)
        n1644 = local read "DISPLACEMENT : 4"() -> (w2261:dbl)
        n1645 = local read "TEMPERATURE : 2"() -> (w2259:dbl)
        n1646 = local read "DISPLACEMENT :"() -> (w2260:dbl)
        n1647 = local read "STROKE GAIN : 2"() -> (w2265:dbl)
        n1648 = local read "FRIC. FORCE : 2"() -> (w2268:dbl)
        n1649 = local read "TEMPERATURE :"() -> (w2257:dbl)
        n1650 = local read "STROKE GAIN :"() -> (w2264:dbl)
        n1651 = local read "FRIC. FORCE :"() -> (w2267:dbl)
        n1652 = stacked-sequence {
          frame #0 {
            n1653 = local read "EDIT"() -> (w2298:bool)
            n1654 = case shown="True" w2298 {
              tunnel: [u8 2 ("Disabled") u8 0 ("Disabled")] -> _
              frame False {
                w2300 = FALSE
                n1655 = local write "Password"("") -> ()
                n1656 = property on="message" class="Str"("Visible"=w2300) -> ()  [unwired: 2 in, 2 out]
                n1657 = local write "x = y?"(w2300) -> ()
                n1658 = property on="SrvM CP" class="Bool (strict)"("Visible"=w2300) -> ()  [unwired: 2 in, 2 out]
                n1659 = property on="Password" class="Str"("Visible"=w2300) -> ()  [unwired: 2 in, 2 out]
                n1660 = local write "SrvM CP"(w2300) -> ()
                n1661 = property on="ENTER THE NEW PASSWORD" class="Str"("Visible"=w2300) -> ()  [unwired: 2 in, 2 out]
                n1662 = property on="ENTER CURRENT PASSWORD" class="Str"("Visible"=w2300) -> ()  [unwired: 2 in, 2 out]
              }
              frame True {
                w2303 = TRUE
                n1663 = property on="SrvM CP" class="Bool (strict)"("Visible"=w2303) -> ()  [unwired: 2 in, 2 out]
                n1664 = property on="Password" class="Str"("Visible"=w2303) -> ()  [unwired: 2 in, 2 out]
              }
            }
            "dipl pwd" <- "@143$\n" ("dipl pwd")
          }
          frame #1 {
            # "Gain password"
            n1665 = String To Byte Array(string="ENTER CURRENT PASSWORD") -> (unsigned byte array=w2308:u8[])
            n1666 = Search 1D Array(1D array=w2308, element=u8 10) -> (index of element=w2311:i32)  [unwired: 1 in]
            n1667 = Index Array(array=w2308, index=w2311) -> (element=w2307:u8)
            n1668 = Equal?(x=w2307, y=10) -> (x = y?=w2305:bool)
            n1669 = case shown="True" w2305 {
              frame False {
                n1670 = property on="ENTER THE NEW PASSWORD" class="Str"("Visible"=FALSE) -> ()  [unwired: 2 in, 2 out]
              }
              frame True {
                # "password"
                # "change password logic"
                n1671 = local read "ENTER CURRENT PASSWORD"() -> (w2324:string)
                n1672 = local read "dipl pwd"() -> (w2318:string)
                n1673 = String To Byte Array(string=w2318) -> (unsigned byte array=w2319:u8[])
                n1674 = String To Byte Array(string=w2324) -> (unsigned byte array=w2326:u8[])
                n1675 = Array Size(array=w2319) -> (size(s)=w2321:i32)
                n1676 = Array Size(array=w2326) -> (size(s)=w2323:i32)
                n1677 = for {
                  N: w2321 -> [_]
                  tunnel: w2319 -> [w2338]
                  tunnel: [w2336] -> w2320 mode=indexing
                  tunnel: w2321 -> [w2333]
                  i -> [w2334]
                  n1678 = Decrement(x=w2333) -> (x-1=w2332:i32)
                  n1679 = Equal?(x=w2334, y=w2332) -> (x = y?=w2331:bool)
                  n1680 = Index Array(array=w2338, index=w2334) -> (element=w2337:u8)
                  n1681 = Number To Decimal String(number=w2337) -> (decimal integer string=w2335:string)  [unwired: 1 in]
                  n1682 = Select(t="", s=w2331, f="\r") -> (s? t:f=w2328:string)
                  n1683 = Concatenate Strings(w2335, w2328) -> (w2336:string)
                }
                n1684 = for {
                  N: w2323 -> [_]
                  tunnel: w2326 -> [w2350]
                  tunnel: [w2348] -> w2327 mode=indexing
                  tunnel: w2323 -> [w2342]
                  i -> [w2343]
                  n1685 = Decrement(x=w2342) -> (x-1=w2340:i32)
                  n1686 = Equal?(x=w2343, y=w2340) -> (x = y?=w2341:bool)
                  n1687 = Index Array(array=w2350, index=w2343) -> (element=w2344:u8)
                  n1688 = Number To Decimal String(number=w2344) -> (decimal integer string=w2349:string)  [unwired: 1 in]
                  n1689 = Select(t="", s=w2341, f="\r") -> (s? t:f=w2346:string)
                  n1690 = Concatenate Strings(w2349, w2346) -> (w2348:string)
                }
                n1691 = local read "string"() -> (w2325:string)
                n1692 = Concatenate Strings(w2320) -> (w2314:string)
                n1693 = Concatenate Strings(w2325) -> (w2322:string)
                n1694 = Concatenate Strings(w2327) -> (w2315:string)
                n1695 = Equal?(x=w2315, y=w2314) -> (x = y?=w2313:bool)
                n1696 = Equal?(x=w2315, y=w2322) -> (x = y?=w2317:bool)
                n1697 = Or(x=w2317, y=w2313) -> (x .or. y?=w2316:bool)
                n1698 = case shown="True" w2316 {
                  frame False {
                  }
                  frame True {
                    n1699 = property on="ENTER THE NEW PASSWORD" class="Str"("Visible"=TRUE) -> ()  [unwired: 2 in, 2 out]
                  }
                }
              }
            }
          }
          frame #2 {
            n1700 = String To Byte Array(string="ENTER THE NEW PASSWORD") -> (unsigned byte array=w2353:u8[])
            n1701 = Search 1D Array(1D array=w2353, element=u8 10) -> (index of element=w2357:i32)  [unwired: 1 in]
            n1702 = Index Array(array=w2353, index=w2357) -> (element=w2355:u8)
            n1703 = Equal?(x=w2355, y=10) -> (x = y?=w2352:bool)
            n1704 = case shown="False" w2352 {
              frame False {
              }
              frame True {
                n1705 = local write "EDIT"(FALSE) -> ()
                n1706 = local write "SrvM CP"(FALSE) -> ()
                n1707 = local read "ENTER THE NEW PASSWORD"() -> (w2360:string)
                n1708 = String To Byte Array(string=w2360) -> (unsigned byte array=w2365:u8[])
                n1709 = Array Size(array=w2365) -> (size(s)=w2362:i32)
                n1710 = for {
                  N: w2362 -> [_]
                  tunnel: w2365 -> [w2378]
                  tunnel: [w2375] -> w2367 mode=indexing
                  tunnel: w2362 -> [w2370]
                  i -> [w2368]
                  n1711 = Decrement(x=w2370) -> (x-1=w2371:i32)
                  n1712 = Equal?(x=w2368, y=w2371) -> (x = y?=w2372:bool)
                  n1713 = Index Array(array=w2378, index=w2368) -> (element=w2377:u8)
                  n1714 = Number To Decimal String(number=w2377) -> (decimal integer string=w2376:string)  [unwired: 1 in]
                  n1715 = Select(t="", s=w2372, f="\r") -> (s? t:f=w2369:string)
                  n1716 = Concatenate Strings(w2376, w2369) -> (w2375:string)
                }
                n1717 = local read "file path"() -> (w2359:path)
                n1718 = Concatenate Strings(w2367) -> (w2361:string)
                n1719 = Delete(path (use dialog)=w2359) -> (deleted path=w2363:path)  [unwired: 4 in, 2 out]
                n1720 = call <vilib>:"Write Characters To File.vi"("append to file? (new file:F)"=FALSE, "character string"=w2361, "file path (dialog if empty)"=w2363) -> ()  [unwired: 2 in, 1 out]
              }
            }
          }
          frame #3 {
            n1721 = case shown="True" "SrvM CP" {
              frame False {
                w2381 = ""
                n1722 = property on="ENTER CURRENT PASSWORD" class="Str"("Visible"=FALSE) -> ()  [unwired: 2 in, 2 out]
                n1723 = local write "ENTER THE NEW PASSWORD"(w2381) -> ()
                n1724 = local write "ENTER CURRENT PASSWORD"(w2381) -> ()
              }
              frame True {
                n1725 = property on="ENTER THE NEW PASSWORD" class="Str"() -> ("Visible"=w2382:bool)  [unwired: 2 in, 2 out]
                n1726 = Not(x=w2382) -> (.not. x?=w2383:bool)
                n1727 = property on="ENTER CURRENT PASSWORD" class="Str"("Visible"=w2383) -> ()  [unwired: 2 in, 2 out]
              }
            }
          }
          frame #4 {
            n1728 = String To Byte Array(string="Password") -> (unsigned byte array=w2390:u8[])
            n1729 = Search 1D Array(1D array=w2390, element=u8 10) -> (index of element=w2388:i32)  [unwired: 1 in]
            n1730 = Index Array(array=w2390, index=w2388) -> (element=w2389:u8)
            n1731 = Equal?(x=w2389, y=10) -> (x = y?=w2385:bool)
            n1732 = case shown="True" w2385 {
              frame False {
              }
              frame True {
                # "password"
                # "password"
                n1733 = local read "Password"() -> (w2403:string)
                n1734 = String To Byte Array(string="@143$\n") -> (unsigned byte array=w2392:u8[])
                n1735 = String To Byte Array(string=w2403) -> (unsigned byte array=w2406:u8[])
                n1736 = Array Size(array=w2392) -> (size(s)=w2397:i32)
                n1737 = Array Size(array=w2406) -> (size(s)=w2401:i32)
                n1738 = for {
                  N: w2401 -> [_]
                  tunnel: w2406 -> [w2440]
                  tunnel: [w2438] -> w2407 mode=indexing
                  tunnel: w2401 -> [w2435]
                  i -> [w2436]
                  n1739 = Decrement(x=w2435) -> (x-1=w2434:i32)
                  n1740 = Equal?(x=w2436, y=w2434) -> (x = y?=w2433:bool)
                  n1741 = Index Array(array=w2440, index=w2436) -> (element=w2439:u8)
                  n1742 = Number To Decimal String(number=w2439) -> (decimal integer string=w2437:string)  [unwired: 1 in]
                  n1743 = Select(t="", s=w2433, f="\r") -> (s? t:f=w2430:string)
                  n1744 = Concatenate Strings(w2437, w2430) -> (w2438:string)
                }
                n1745 = for {
                  N: w2397 -> [_]
                  tunnel: w2392 -> [w2451]
                  tunnel: [w2449] -> w2395 mode=indexing
                  tunnel: w2397 -> [w2446]
                  i -> [w2447]
                  n1746 = Decrement(x=w2446) -> (x-1=w2445:i32)
                  n1747 = Equal?(x=w2447, y=w2445) -> (x = y?=w2444:bool)
                  n1748 = Index Array(array=w2451, index=w2447) -> (element=w2450:u8)
                  n1749 = Number To Decimal String(number=w2450) -> (decimal integer string=w2448:string)  [unwired: 1 in]
                  n1750 = Select(t="", s=w2444, f="\r") -> (s? t:f=w2441:string)
                  n1751 = Concatenate Strings(w2448, w2441) -> (w2449:string)
                }
                n1752 = local read "file path"() -> (w2391:path)
                n1753 = call <vilib>:"Read Characters From File.vi"("file path (dialog if empty)"=w2391) -> ("character string"=w2405:string)  [unwired: 5 in, 3 out]
                "string" <- w2405
                n1754 = flat-sequence {
                  tunnel: [w2408] -> w2402
                  frame #0 {
                    w2408 = ""
                    n1755 = local write "Password"(w2408) -> ()
                  }
                }
                n1756 = Concatenate Strings(w2395) -> (w2396:string)
                n1757 = Concatenate Strings(w2405) -> (w2404:string)
                n1758 = Concatenate Strings(w2407) -> (w2399:string)
                n1759 = Equal?(x=w2399, y=w2396) -> (x = y?=w2400:bool)
                n1760 = Equal?(x=w2399, y=w2404) -> (x = y?=w2394:bool)
                n1761 = Or(x=w2394, y=w2400) -> (x .or. y?=w2393:bool)
                "x = y?" <- w2393
                n1762 = case shown="True" w2393 {
                  selector: w2393 -> [w2410 _]
                  tunnel: w2402 -> [_ _]
                  frame False {
                    n1763 = And(x=w2410, y=TRUE ("Visible")) -> (x .and. y?=w2411:bool)
                    n1764 = property on="message" class="Str"("Visible"=w2411) -> ()  [unwired: 2 in, 2 out]
                  }
                  frame True {
                    n1765 = control-ref of="This VI"() -> (w2422:refnum<vi>)
                    n1766 = property class="VI"(reference=w2422) -> (reference out=w2413:refnum<vi>, error out=w2417:errorcluster, "Panel"=w2421:refnum<vi>)  [unwired: 1 in]
                    n1767 = property on="message" class="Str"("Visible"=FALSE) -> ()  [unwired: 2 in, 2 out]
                    n1768 = property class="Pnl"(reference=w2421, error in=w2417) -> (reference out=w2415:refnum<vi>, error out=w2418:errorcluster, "Panes[]"=w2420:refnum<vi>[])
                    n1769 = for {
                      tunnel: w2420 -> [w2429] mode=indexing
                      tunnel: T18."Always On" ("Horizontal Scrollbar Visibility") -> [w2428]
                      tunnel: w2418 -> [w2425]
                      tunnel: [w2424] -> w2416
                      n1770 = property class="Pane"(reference=w2429, error in=w2425, "HorizScrollbarVisibility"=w2428) -> (reference out=w2426:refnum<vi>, error out=w2427:errorcluster)
                      n1771 = Close Reference(reference=w2426, error in (no error)=w2427) -> (error out=w2424:errorcluster)
                    }
                    n1772 = Close Reference(reference=w2415, error in (no error)=w2416) -> (error out=w2414:errorcluster)
                    n1773 = Close Reference(reference=w2413, error in (no error)=w2414) -> (error out=→"error out 6":errorcluster)
                  }
                }
              }
            }
          }
        }
        n1774 = case shown="True" w2248 {
          tunnel: [u8 2 ("Disabled") u8 0 ("Disabled")] -> w2247
          tunnel: [w2612 TRUE ("Visible")] -> w2246
          frame False {
            w2612 = FALSE ("Visible")
            n1775 = local write "EDIT 2"(w2612) -> ()
          }
          frame True {
          }
        }
        n1776 = Subtract(x=w2252, y=w2251) -> (x-y=w2253:dbl)
        n1777 = local read "AIR TEMPERATURE : 2"() -> (w2256:dbl)
        n1778 = local read "AIR TEMPERATURE :"() -> (w2255:dbl)
        n1779 = Subtract(x=w2259, y=w2257) -> (x-y=w2258:dbl)
        n1780 = Subtract(x=w2261, y=w2260) -> (x-y=w2262:dbl)
        n1781 = Subtract(x=w2265, y=w2264) -> (x-y=w2263:dbl)
        n1782 = Subtract(x=w2268, y=w2267) -> (x-y=w2266:dbl)
        n1783 = Divide(x=w2253, y=w2251) -> (x/y=w2275:dbl)
        n1784 = Subtract(x=w2256, y=w2255) -> (x-y=w2254:dbl)
        n1785 = Divide(x=w2258, y=w2257) -> (x/y=w2279:dbl)
        n1786 = Divide(x=w2262, y=w2260) -> (x/y=w2282:dbl)
        n1787 = Divide(x=w2263, y=w2264) -> (x/y=w2283:dbl)
        n1788 = Divide(x=w2266, y=w2267) -> (x/y=w2286:dbl)
        n1789 = Multiply(x=w2275, y=100.0) -> (x*y=→"HUMIDITY  Calibration Error":dbl)
        n1790 = Divide(x=w2254, y=w2255) -> (x/y=w2278:dbl)
        n1791 = Multiply(x=w2279, y=100.0) -> (x*y=→"TEMPERATURE  Calibration Error":dbl)
        n1792 = Multiply(x=w2282, y=100.0) -> (x*y=→"DISPLACEMENT  Calibration Error":dbl)
        n1793 = Multiply(x=w2283, y=100.0) -> (x*y=→"STROKE Calibration Error":dbl)
        n1794 = Multiply(x=w2286, y=100.0) -> (x*y=→"FRIC. FORCE Calibration Error":dbl)
        n1795 = property on="EDIT 2" class="Bool (strict)"("Visible"=w2246) -> ()  [unwired: 2 in, 2 out]
        n1796 = property on="SrvM CP" class="Bool (strict)"("Disabled"=w2247) -> ()  [unwired: 2 in, 2 out]
        n1797 = property on="File Path" class="Path"("Disabled"=w2247) -> ()  [unwired: 2 in, 2 out]
        n1798 = property on="visa due" class="CmbBox"("Disabled"=w2247) -> ()  [unwired: 2 in, 2 out]
        n1799 = property on="SAVE" class="Bool (strict)"("Visible"=w2246) -> ()  [unwired: 2 in, 2 out]
        n1800 = Multiply(x=w2278, y=100.0) -> (x*y=→"AIR TEMPERATURE  Calibration Error":dbl)
        n1801 = case shown="True" w2245 {
          frame False {
          }
          frame True {
            n1802 = stacked-sequence {
              seq-local: [w2460 _ _] -> [_ w2607 _]
              frame #0 {
                (unwired) i16 5 ("precision (6)")
                # "[CH1]    - FF\n[CH2]   - TEMPERATURE\n[CH3]    - Humidity\n[CH4]    - AIR TEMP\n[CH5]\\- Visa Uno\n[CH6] \\- Visa Due\n[CH7]  \\- file path\n[CH8]   - Displacement Gain\n[CHA]   - Stroke Gain\n[CHB]   - Stroke PID Gain\n[CHC]   -Language Selection\n[CHD]   -Power +\n[CHE]   -Power_\n[CHF]   -Heater\n[CHG]   -Humidity Wet\n[CHH]   -Humidity Dry\n[CHI]   -Integral Time"
                n1803 = local read "Language Selection"() -> (w2508:enum16{"English", "Russian"})
                n1804 = local read "CH-HUMIDITY WET"() -> (w2466:u16)
                n1805 = local read "CH-HUMIDITY DRY"() -> (w2463:u16)
                n1806 = local read "STROKE GAIN :"() -> (w2452:dbl)
                n1807 = local read "CH-POWER +"() -> (w2475:u16)
                n1808 = local read "CH-POWER -"() -> (w2472:u16)
                n1809 = local read "CH-HEATER"() -> (w2469:u16)
                n1810 = local read "AIR TEMPERATURE :"() -> (w2455:dbl)
                n1811 = local read "DISPLACEMENT :"() -> (w2453:dbl)
